vi "Calculate Mean and Standard Deviation.vi"(11 "Statistics in":refnum<class "JSON Value.lvclass">) -> (3 "Mean and Standard Deviation(SD)":refnum<class "JSON Value.lvclass">)   [LabVIEW 2020, in "Library Commun.lvlib" / "JSON Statistics.lvclass"]
uses:
  JSON Statistics.lvclass
  JSON Value/JSON Value.lvclass
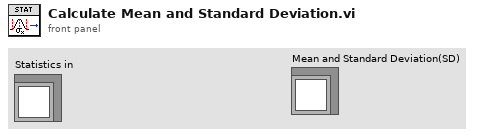
[diagram p1: front panel]
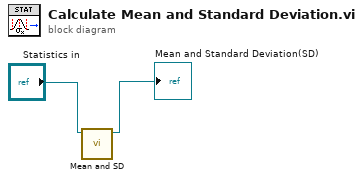
[diagram p0: block diagram]
diagram:
  n1 = call-dynamic "Mean and SD.vi"("Statistics in"="Statistics in") -> ("Mean and Standard Deviation(SD)"=→"Mean and Standard Deviation(SD)":refnum<class "JSON Value.lvclass">)  [unwired: 8 in, 2 out]
